vi "init_tour_in_progress.vi"(1 "starting_square":T1) -> (0 "blank_tour_in_progress":T2)   [LabVIEW 2020, in "core.lvlib"]
uses:
  core.lvlib
  core_data/tour_in_progress.ctl
  core_data/chessboard_index.ctl
  core_data/core_data.lvlib
panel:
  # "Development\ncontrols/indicators useful for development and testing, but which are not outputs of the VI"
  # "Input\nInputs to the VI"
  # "Output\nOutputs of the VI"
  # "Description\n\nBlank VI with error handling case. \n\nSummarize the use of this VI in this space."
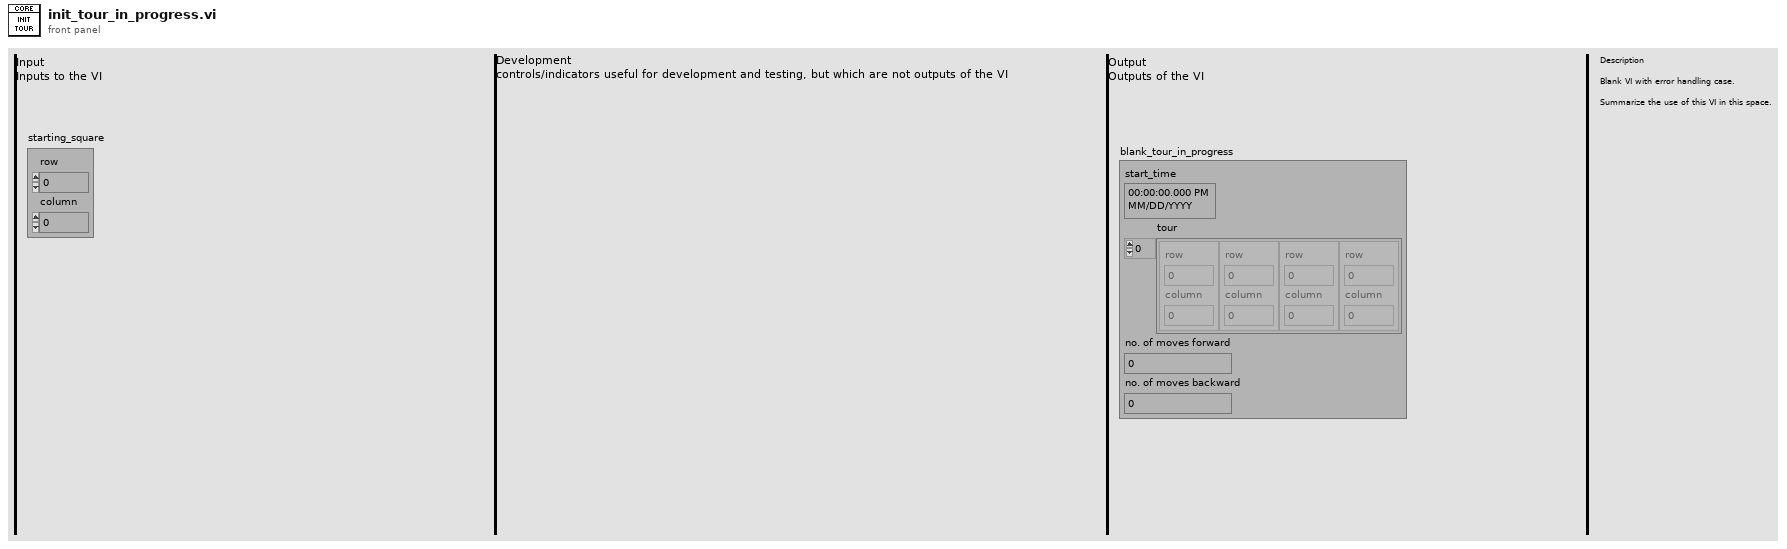
[diagram p1: front panel]
types:
  T1 = typedef "core.lvlib/core_data.lvlib/chessboard_index.ctl" = cluster{"row":u8, "column":u8}
  T2 = typedef "core.lvlib/core_data.lvlib/tour_in_progress.ctl" = cluster{"start_time":timestamp, "tour":T1[], "no. of moves forward":u64, "no. of moves backward":u64}
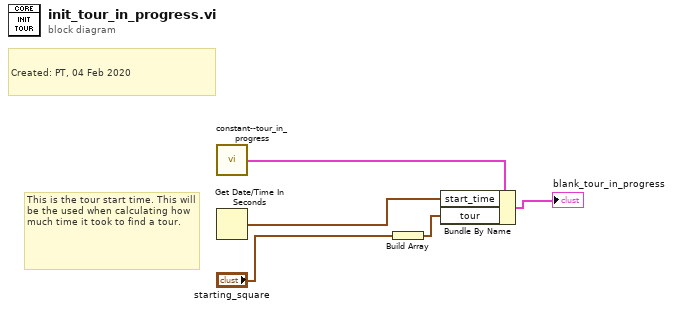
[diagram p0: block diagram]
diagram:
  # "This is the tour start time. This will be the used when calculating how much time it took to find a tour."
  # "Created: PT, 04 Feb 2020"
  n1 = call "constant--tour_in_progress.vi"() -> ("blank_tour_in_progress"=w3:T2)
  n2 = Get Date/Time In Seconds() -> (seconds since 1Jan1904=w2:timestamp)
  n3 = Build Array("starting_square") -> (w1:T1[])
  n4 = Bundle By Name(cluster=w3, "start_time"=w2, "tour"=w1) -> (→"blank_tour_in_progress":T2)
